vi "EstimateTransformParametersBetweenPointSets.vi"(7 "Fix Scale at 1.0?":bool, 8 "error in":errorcluster, 9 "To Point Set":T2, 11 "From Point Set":T2) -> (0 "error out":errorcluster, 1 "c":dbl, 2 "t":dbl[](array[numeric]), 3 "R":T1, 4 "Minimum Mean Square Error":dbl)   [LabVIEW 2020, in "ar.lvlib"]
uses:
  ar.lvlib
  PointSet.ctl
  <vilib>/Analysis/Matrix/Datatypes/RealMatrix.ctl
  <vilib>/Analysis/baseanly.llb/Mean.vi
  <vilib>/Analysis/baseanly.llb/Mean (DBL).vi
  <vilib>/Analysis/baseanly.llb/A x B.vi
  <vilib>/Analysis/baseanly.llb/Real A x B.vi
  <vilib>/Analysis/baseanly.llb/Determinant.vi
  <vilib>/Analysis/baseanly.llb/Real Determinant.vi
  SVDForPointSetCovarainces.vi
  <vilib>/Analysis/_algsub.llb/Matrix Rank.vi
  <vilib>/Analysis/_algsub.llb/Real Matrix Rank.vi
  <vilib>/Analysis/_algsub.llb/Trace.vi
  <vilib>/Analysis/_algsub.llb/Real Matrix Trace.vi
  <vilib>/Utility/error.llb/Error Cluster From Error Code.vi
  <vilib>/Analysis/Matrix/Numeric/Conversions/Array To Matrix - RA2.vi
  <vilib>/Analysis/7linalg.llb/SVD Decomposition.vi
  <vilib>/Analysis/7linalg.llb/Real SVD Decomposition.vi
  <vilib>/Analysis/7linalg.llb/Create Special Matrix.vi
  <vilib>/Analysis/7linalg.llb/Create Special Real Matrix.vi
  <vilib>/ErrorRing/Error Ring.xnode
  <vilib>/Analysis/NI_AALBase.lvlib
  <vilib>/Analysis/Matrix/NI_Matrix.lvlib
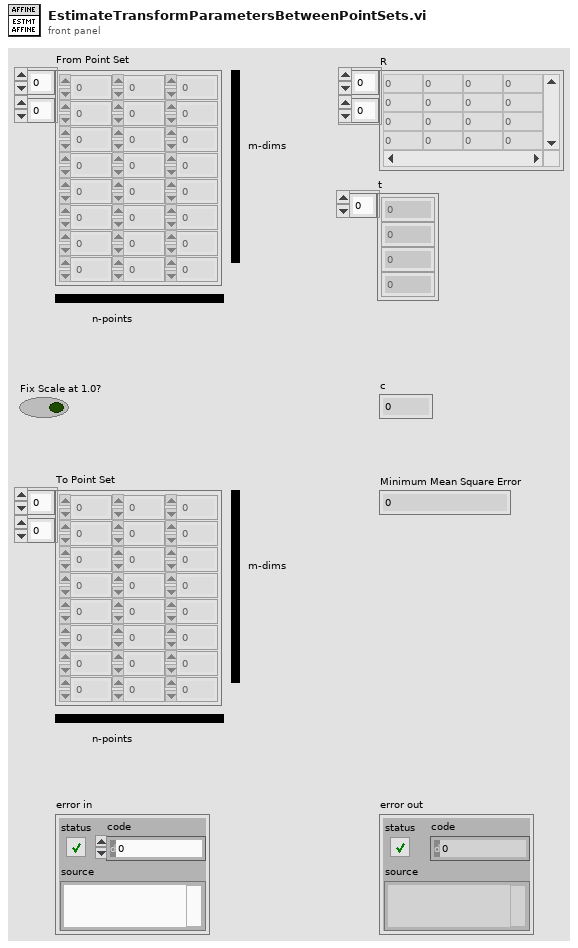
[diagram p1: front panel]
types:
  T1 = typedef "NI_Matrix.lvlib/RealMatrix.ctl" = dbl[][]
  T2 = typedef "ar.lvlib/PointSet.ctl" = dbl[][]
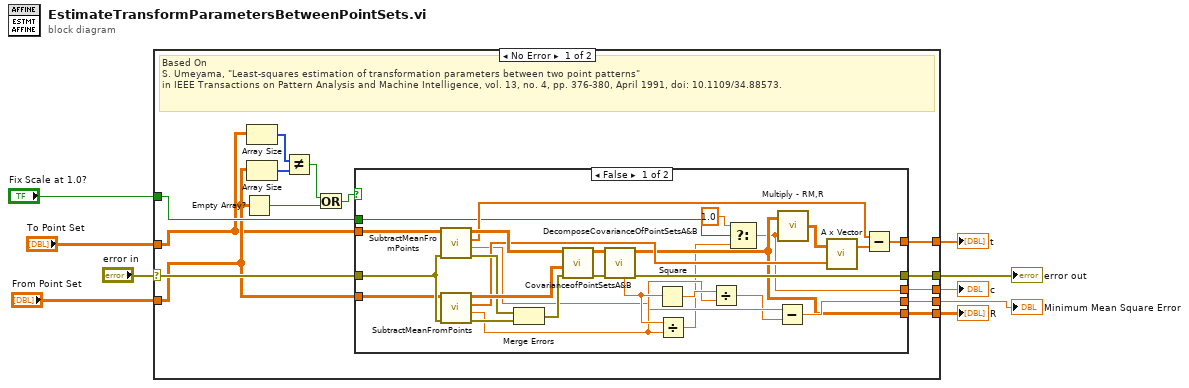
[diagram p0: block diagram]
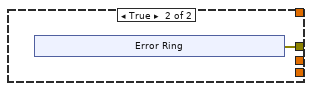
[diagram p2: hidden frame]
diagram:
  n1 = case shown="No Error" "error in" {
    selector: "error in" -> [w22 w57]
    tunnel: "To Point Set" -> [w12 _]
    tunnel: "From Point Set" -> [w13 _]
    tunnel: [w23 w57] -> w8
    tunnel: [w21 _] -> w7
    tunnel: [w18 _] -> w6
    tunnel: [w20 _] -> w5
    tunnel: [w19 _] -> w4
    tunnel: "Fix Scale at 1.0?" -> [w17 _]
    frame No Error {
      # "Based On\nS. Umeyama, \"Least-squares estimation of transformation parameters between two point patterns\" \nin IEEE Transactions on Pattern Analysis and Machine Intelligence, vol. 13, no. 4, pp. 376-380, April 1991, doi: 10.1109/34.88573."
      n2 = Empty Array?(array=w13) -> (empty?=w16:bool)
      n3 = Array Size(array=w12) -> (size(s)=w11:i32[])
      n4 = Array Size(array=w13) -> (size(s)=w14:i32[])
      n5 = Not Equal?(x=w11, y=w14) -> (x != y?=w15:bool)
      n6 = Or(x=w15, y=w16) -> (x .or. y?=w10:bool)
      n7 = case shown="False" w10 {
        tunnel: [w49 w51] -> w23
        tunnel: w22 -> [w39 _]
        tunnel: [w32 _] -> w21
        tunnel: [w31 _] -> w20
        tunnel: [w30 _] -> w19
        tunnel: [w28 _] -> w18
        tunnel: w17 -> [w26 _]
        tunnel: w13 -> [w25 _]
        tunnel: w12 -> [w24 _]
        frame False {
          n8 = call "SubtractMeanFromPoints.vi"("error in"=w39, "x"=w24) -> ("error out"=w45:errorcluster, "var(x)"=w34:dbl, "mean(x)"=w40:dbl[], "x - mean(x)"=w50:dbl[][])  [unwired: 6 in]
          n9 = call "SubtractMeanFromPoints.vi"("error in"=w39, "x"=w25) -> ("error out"=w47:errorcluster, "var(x)"=w35:dbl, "mean(x)"=w42:dbl[], "x - mean(x)"=w48:dbl[][])  [unwired: 6 in]
          n10 = Merge Errors(w45, w47) -> (w46:errorcluster)
          n11 = call "CovarianceofPointSetsA&B.vi"("error in (no error)"=w46, "A - mean(A)"=w48, "B - mean(B)"=w50) -> ("error out"=w38:errorcluster, "Covariance"=w44:T1)  [unwired: 7 in]
          n12 = call "DecomposeCovarianceOfPointSetsA&B.vi"("error in (no error)"=w38, "Covariance A & B"=w44) -> ("error out"=w49:errorcluster, "R"=w31:T1, "Trace(DS)"=w37:dbl)  [unwired: 7 in]
          n13 = Square(x=w37) -> (x^2=w36:dbl)
          n14 = Divide(x=w37, y=w35) -> (x/y=w29:dbl)
          n15 = Divide(x=w36, y=w35) -> (x/y=w33:dbl)
          n16 = Select(t=1.0 ("f"), s=w26, f=w29) -> (s? t:f=w28:dbl)
          n17 = Subtract(x=w34, y=w33) -> (x-y=w32:dbl)
          n18 = call <vilib>:"Multiply - RM,R.vi"("Real Scalar c"=w28, "Real Matrix A"=w31) -> ("A * c"=w43:T1)
          n19 = call <vilib>:"A x Vector.vi"("Vector"=w42, "A"=w43) -> ("A x Vector"=w41:dbl[])  [unwired: 1 out]
          n20 = Subtract(x=w40, y=w41) -> (x-y=w30:dbl[])
        }
        frame True {
          n21 = xnode "Error Ring"() -> ("error out"=w51:errorcluster)
        }
      }
    }
    frame Error {
    }
  }
  "error out" <- w8
  "Minimum Mean Square Error" <- w7
  "c" <- w6
  "R" <- w5
  "t" <- w4
